vi "Initialise.vi"(8 "error in (no error)":errorcluster, 11 "Actor in":refnum<class "Error Handler Actor.lvclass">) -> (0 "error out":errorcluster, 3 "Actor out":refnum<class "Error Handler Actor.lvclass">, 5 "Observers":cluster{"Actor":refnum<event-registration>})   [LabVIEW 2021, in "Error Handler Actor.lvclass"]
uses:
  Error Handler Actor.lvclass
  Error Handler Actor.lvclass/Error Handler Actor.ctl
  Re-use Libraries/Utility/Utility.lvlib
  Re-use Libraries/Minimal Actor Framework/Messaging/Message/Message.lvclass
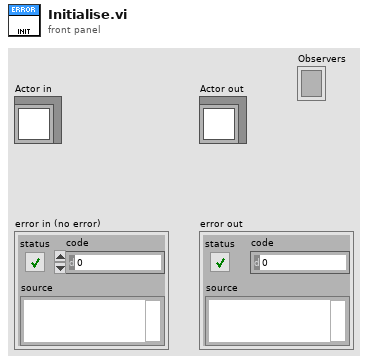
[diagram p1: front panel]
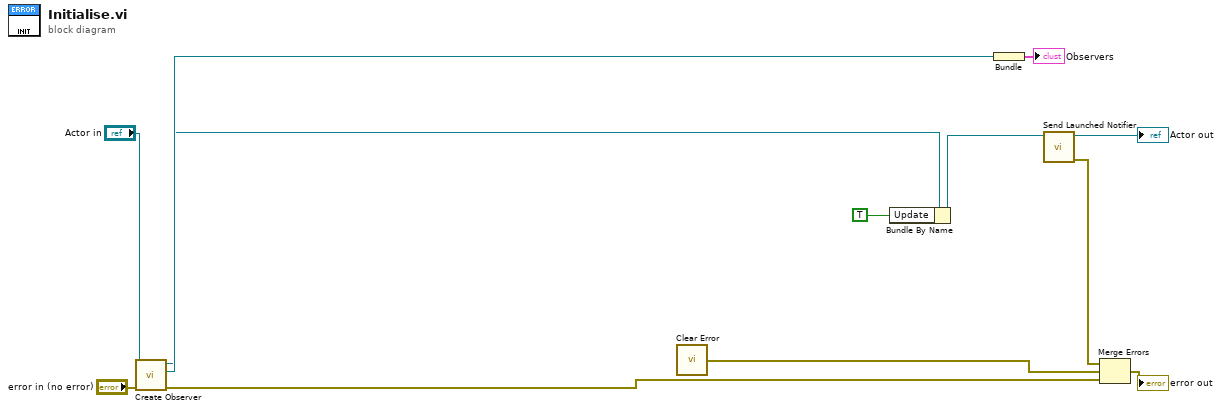
[diagram p0: block diagram]
diagram:
  n1 = call-dynamic "Create Observer.vi"("error in (no error)"="error in (no error)", "Actor in"="Actor in") -> ("error out"=w3:errorcluster, "Actor"=w6:refnum<event-registration>, "Actor out"=w5:refnum<class "Error Handler Actor.lvclass">)  [unwired: 7 in]
  n2 = call "Clear Error.vi"() -> ("error out"=w2:errorcluster)  [unwired: 1 in]
  n3 = Bundle By Name(cluster=w5, "Update"=TRUE) -> (w9:refnum<class "Error Handler Actor.lvclass">)
  n4 = Bundle("Actor"=w6) -> (→"Observers":cluster{"Actor":refnum<event-registration>})  [unwired: 1 in]
  n5 = call-dynamic "Send Launched Notifier.vi"("Actor in"=w9) -> ("error out"=w4:errorcluster, "Actor out"=→"Actor out":refnum<class "Error Handler Actor.lvclass">)  [unwired: 9 in]
  n6 = Merge Errors(w4, w2, w3) -> (→"error out":errorcluster)
